vi "Global 2.vi"() -> ()   [LabVIEW 2014]
panel:
  in  "A":waveform(dbl)[](array[waveform])
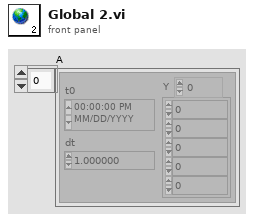
[diagram p1: front panel]
diagram:
